vi "Format System Configuration Log.vi"(8 "error in (no error)":errorcluster, 11 "Instrument.Lockin in":refnum<class "Instrument.Lockin.lvclass">) -> (0 "error out":errorcluster, 1 "System Configuration":T1[](array[typedef]), 2 "Paths":string, 3 "Instrument.Lockin out":refnum<class "Instrument.Lockin.lvclass">, 4 "Times":timestamp[](array[timestamp]))   [LabVIEW 2019, in "Instrument.Lockin.lvlib" / "Instrument.Lockin.lvclass"]
uses:
  Instrument.Lockin.lvclass
  Typedefs/Lockin.LogConfiguration.System--Cluster.ctl
  Instrument.Lockin.lvclass/Instrument.Lockin.ctl
  e44dbd1f-20e5-42cd-913c-705d089ecaef.vi
  39bf8a78-ce5a-4110-a048-be226709f35d.vi
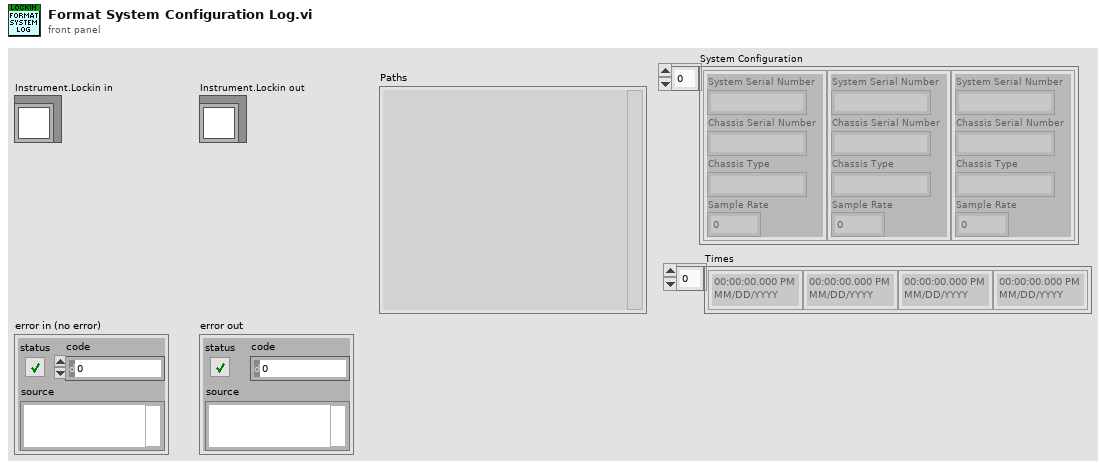
[diagram p1: front panel]
types:
  T1 = typedef "Instrument.Lockin.lvlib/Instrument.Lockin.lvclass/Lockin.LogConfiguration.System--Cluster.ctl" = cluster{"System Serial Number":string, "Chassis Serial Number":string, "Chassis Type":string, "Sample Rate":dbl}
  T2 = typedef "Instrument.Lockin.lvlib/Instrument.DAQ.lvclass/DeviceInfo--Cluster.ctl" = cluster{"DeviceName":string, "DevIsSimulated":bool, "DeviceSerialNumber":string, "ProductType":string, "ProductCategory":i32, "ProductNumber":u32, "ChassisNumber":u32, "SlotNumber":u32, "ChassisName":string, "ChassisSerialNumber":string, "DevTemp":dbl, "SelfCal.LastDate/Time":string, "SelfCal.LastTemp":dbl, "calibration due?":bool}
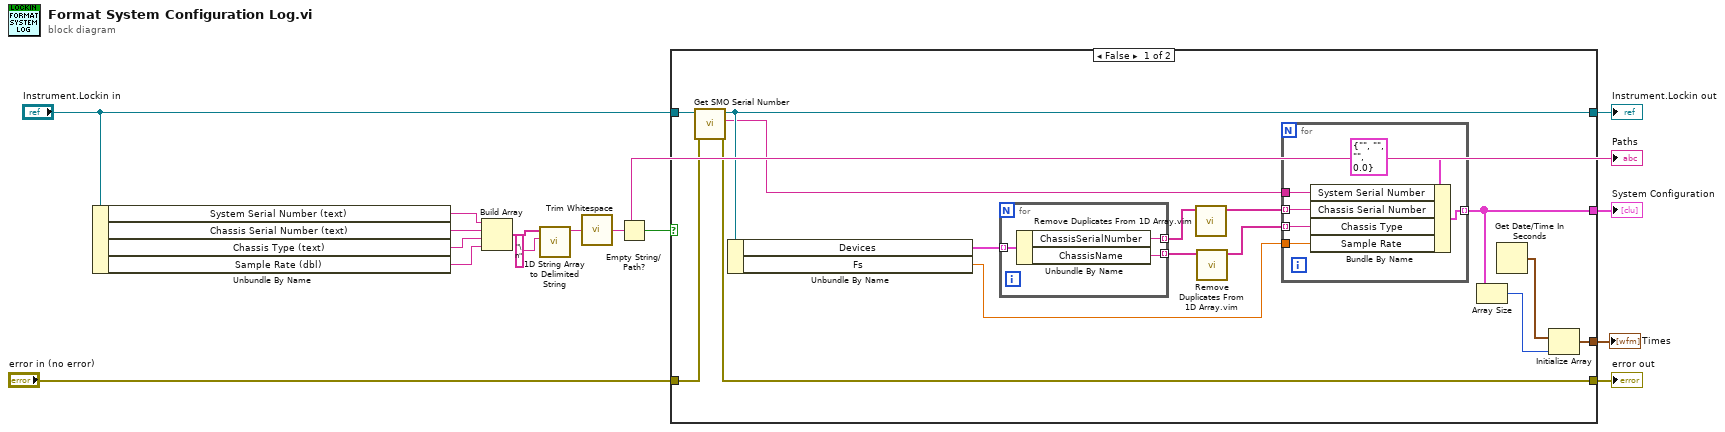
[diagram p0: block diagram]
diagram:
  n1 = Unbundle By Name("Instrument.Lockin in") -> ("System Serial Number (text)"=w9:string, "Chassis Serial Number (text)"=w8:string, "Chassis Type (text)"=w2:string, "Sample Rate (dbl)"=w1:string)
  n2 = Build Array(w9, w8, w2, w1) -> (w7:string[])
  n3 = call <vilib>:"1D String Array to Delimited String.vi"("delimiter"="\n", "string array"=w7) -> ("delimited string"=w10:string)  [unwired: 9 in]
  n4 = call <vilib>:"Trim Whitespace.vi"("string"=w10) -> ("trimmed string"=w4:string)  [unwired: 1 in]
  "Paths" <- w4
  n5 = Empty String/Path?(string/path=w4) -> (empty?=w5:bool)
  n6 = case shown="False" w5 {
    tunnel: [w30 w41] -> w15
    tunnel: [w29 w40] -> w14
    tunnel: "error in (no error)" -> [w27 w40]
    tunnel: [w20 _] -> w12
    tunnel: "Instrument.Lockin in" -> [w21 w41]
    tunnel: [w18 _] -> w3
    frame False {
      n7 = call-dynamic "Get SMO Serial Number.vi"("error in (no error)"=w27, "Instrument.Lockin in"=w21) -> ("error out"=w29:errorcluster, "Serial Number"=w22:string, "Instrument.Lockin out"=w30:refnum<class "Instrument.Lockin.lvclass">)  [unwired: 7 in]
      n8 = Unbundle By Name(w30) -> ("Devices"=w28:T2[], "Fs"=w16:dbl)
      n9 = for {
        tunnel: w28 -> [w33] mode=indexing
        tunnel: [w32] -> w26 mode=indexing
        tunnel: [w31] -> w25 mode=indexing
        n10 = Unbundle By Name(w33) -> ("ChassisSerialNumber"=w32:string, "ChassisName"=w31:string)
      }
      n11 = call "Remove Duplicates From 1D Array.vim"("array"=w26) -> ("array with duplicates removed"=w24:string[])  [unwired: 10 in]
      n12 = call "Remove Duplicates From 1D Array.vim"("array"=w25) -> ("array with duplicates removed"=w23:string[])  [unwired: 10 in]
      n13 = for {
        tunnel: [w39] -> w20 mode=indexing
        tunnel: w24 -> [w37] mode=indexing
        tunnel: w23 -> [w36] mode=indexing
        tunnel: w22 -> [w35]
        tunnel: w16 -> [w34]
        n14 = Bundle By Name(cluster=T1 {"System Serial Number"="", "Chassis Serial Number"="", "Chassis Type"="", "Sample Rate"=0.0} ("System Configuration"), "System Serial Number"=w35, "Chassis Serial Number"=w37, "Chassis Type"=w36, "Sample Rate"=w34) -> (w39:T1)
      }
      n15 = Array Size(array=w20) -> (size(s)=w19:i32)
      n16 = Get Date/Time In Seconds() -> (seconds since 1Jan1904=w17:timestamp)
      n17 = Initialize Array(w17, w19) -> (w18:timestamp[])
    }
    frame True {
    }
  }
  "Instrument.Lockin out" <- w15
  "error out" <- w14
  "System Configuration" <- w12
  "Times" <- w3
